vi "WD_Course_Spin_Parameter.vi"(2 "RpmOptionChoose":enum16{"RPM1400", "RPM1600"}(ring), 3 "路径":path) -> (0 "SpeedTime":T1, 1 "PrjFinalSpinTime":T2)   [LabVIEW 2011]
panel:
  out "EXCEL读取":string[][](array[string])
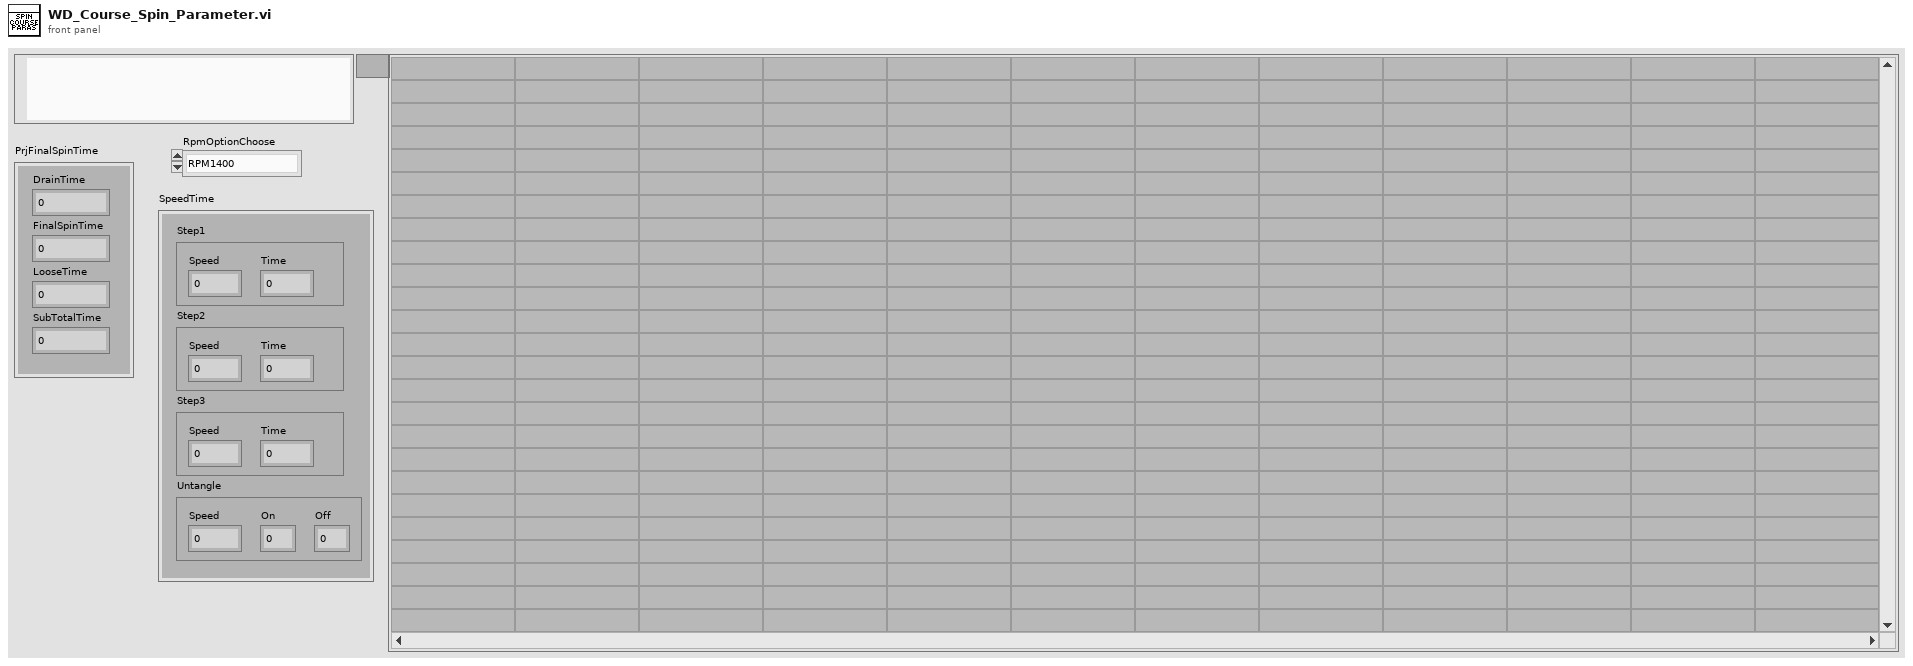
[diagram p1: front panel]
types:
  T1 = cluster{"Step1":cluster{"Speed":u32, "Time":u32}, "Step2":cluster{"Speed":u32, "Time":u32}, "Step3":cluster{"Speed":u32, "Time":u32}, "Untangle":cluster{"Speed":u32, "On":u32, "Off":u32}}
  T2 = cluster{"DrainTime":u32, "FinalSpinTime":u32, "LooseTime":u32, "SubTotalTime":u32}
  T3 = cluster{"Step1":cluster{"Speed":i32, "Time":i32}, "Step2":cluster{"Speed":i32, "Time":i32}, "Step3":cluster{"Speed":i32, "Time":i32}, "Untangle":cluster{"Speed":i32, "On":i32, "Off":i32}}
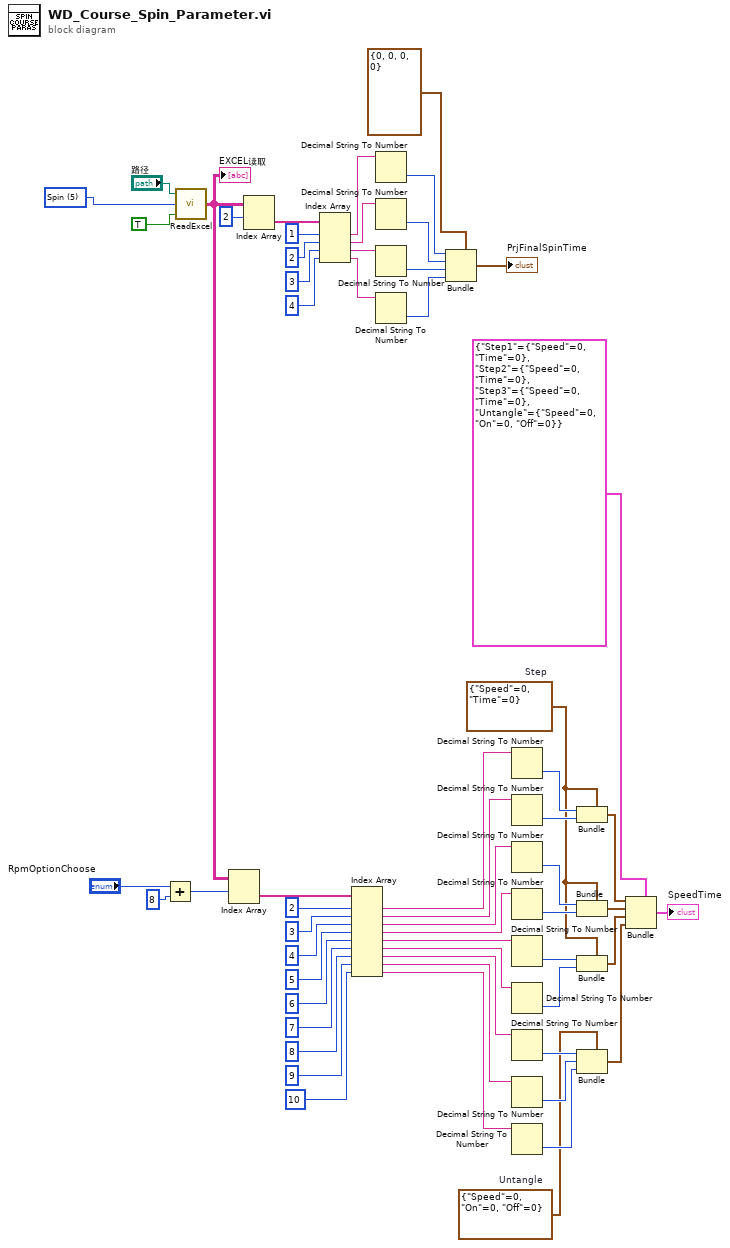
[diagram p0: block diagram]
diagram:
  w1 = u16 5 items=["Init", "Cotton", "eCotton", "Synthetics", "Wool", "Spin", "RinseSpin", "ECPDRUMWASH"]
  w6 = cluster{"Speed":i32, "On":i32, "Off":i32} {"Speed"=0, "On"=0, "Off"=0}  # Untangle
  w7 = cluster{"Speed":i32, "Time":i32} {"Speed"=0, "Time"=0}  # Step
  n1 = Add(x="RpmOptionChoose", y=8 ("索引 (行)")) -> (x+y=w8:i32)
  n2 = call "ReadExcel.vi"("读出文本"=TRUE, "导出sheet位号"=w1, "路径"="路径") -> ("EXCEL读取"=w11:string[][])
  "EXCEL读取" <- w11
  n3 = Index Array(array=w11, index (row)=w8) -> (element=w12:string[])  [unwired: 1 in]
  n4 = Index Array(array=w11, index (row)=2 ("索引 (行)")) -> (element=w56:string[])  [unwired: 1 in]
  n5 = Index Array(array=w56, index #1=1 ("索引"), index #2=2 ("索引"), index #3=3 ("索引"), index #4=4 ("索引")) -> (element #1=w51:string, element #2=w48:string, element #3=w47:string, element #4=w46:string)
  n6 = Index Array(array=w12, index #1=2 ("索引"), index #2=3 ("索引"), index #3=4 ("索引"), index #4=5 ("索引"), index #5=6 ("索引"), index #6=7 ("索引"), index #7=8 ("索引"), index #8=9 ("索引"), index #9=10 ("索引")) -> (element #1=w15:string, element #2=w16:string, element #3=w21:string, element #4=w22:string, element #5=w27:string, element #6=w28:string, element #7=w34:string, element #8=w35:string, element #9=w36:string)
  n7 = Decimal String To Number(string=w51) -> (number=w49:i32)  [unwired: 2 in, 1 out]
  n8 = Decimal String To Number(string=w48) -> (number=w45:i32)  [unwired: 2 in, 1 out]
  n9 = Decimal String To Number(string=w47) -> (number=w44:i32)  [unwired: 2 in, 1 out]
  n10 = Decimal String To Number(string=w46) -> (number=w43:i32)  [unwired: 2 in, 1 out]
  n11 = Bundle(cluster=cluster{i32, i32, i32, i32} {0, 0, 0, 0} ("输入簇"), w49, w45, w44, w43) -> (→"PrjFinalSpinTime":cluster{i32, i32, i32, i32})
  n12 = Decimal String To Number(string=w15) -> (number=w17:i32)  [unwired: 2 in, 1 out]
  n13 = Decimal String To Number(string=w16) -> (number=w18:i32)  [unwired: 2 in, 1 out]
  n14 = Decimal String To Number(string=w21) -> (number=w23:i32)  [unwired: 2 in, 1 out]
  n15 = Decimal String To Number(string=w22) -> (number=w24:i32)  [unwired: 2 in, 1 out]
  n16 = Decimal String To Number(string=w27) -> (number=w30:i32)  [unwired: 2 in, 1 out]
  n17 = Decimal String To Number(string=w28) -> (number=w29:i32)  [unwired: 2 in, 1 out]
  n18 = Decimal String To Number(string=w34) -> (number=w37:i32)  [unwired: 2 in, 1 out]
  n19 = Decimal String To Number(string=w35) -> (number=w38:i32)  [unwired: 2 in, 1 out]
  n20 = Decimal String To Number(string=w36) -> (number=w39:i32)  [unwired: 2 in, 1 out]
  n21 = Bundle(cluster=w7, "Speed"=w17, "Time"=w18) -> (w5:cluster{"Speed":i32, "Time":i32})
  n22 = Bundle(cluster=w7, "Speed"=w23, "Time"=w24) -> (w4:cluster{"Speed":i32, "Time":i32})
  n23 = Bundle(cluster=w7, "Speed"=w30, "Time"=w29) -> (w3:cluster{"Speed":i32, "Time":i32})
  n24 = Bundle(cluster=w6, "Speed"=w37, "On"=w38, "Off"=w39) -> (w2:cluster{"Speed":i32, "On":i32, "Off":i32})
  n25 = Bundle(cluster=T3 {"Step1"={"Speed"=0, "Time"=0}, "Step2"={"Speed"=0, "Time"=0}, "Step3"={"Speed"=0, "Time"=0}, "Untangle"={"Speed"=0, "On"=0, "Off"=0}}, "Step1"=w5, "Step2"=w4, "Step3"=w3, "Untangle"=w2) -> (→"SpeedTime":T3)
